vi "Login_Logout.vi"() -> ()   [LabVIEW 2020]
panel:
  in  "Tab Control":enum32{"Page 1", "Page 2", "Page 3"}(tab)
  in  "Refresh Button":bool
  in  "PassWord":string
  in  "User Name":string
  in  "Port 2":u16
  in  "Port 1":u16
  in  "Stop Send Data":bool
  in  "Send Data Button":bool
  out "Respone Led":bool
  in  "IP address":string
  in  "Export":bool caption="Export data"
  out "data":string[][](array[string]) caption="Data User"
  out "error out":errorcluster
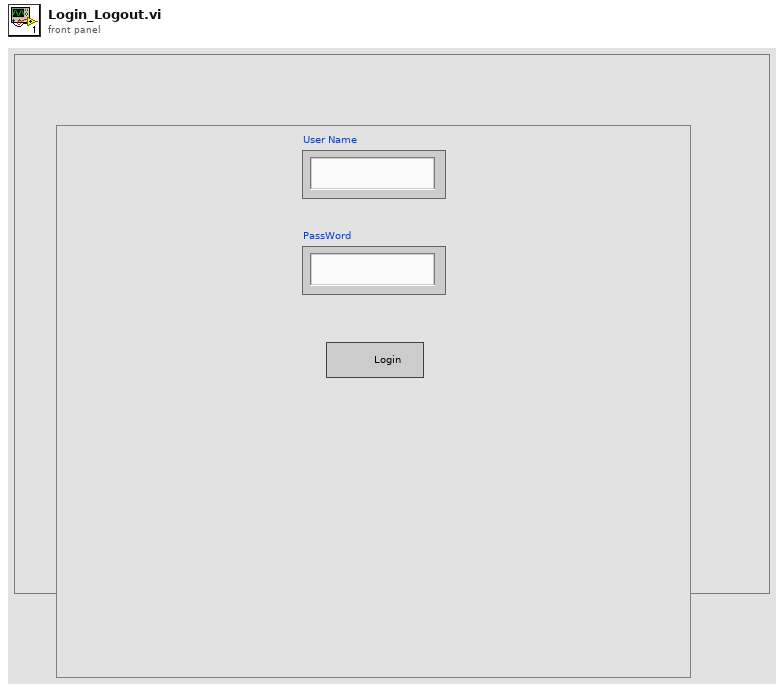
[diagram p1: front panel]
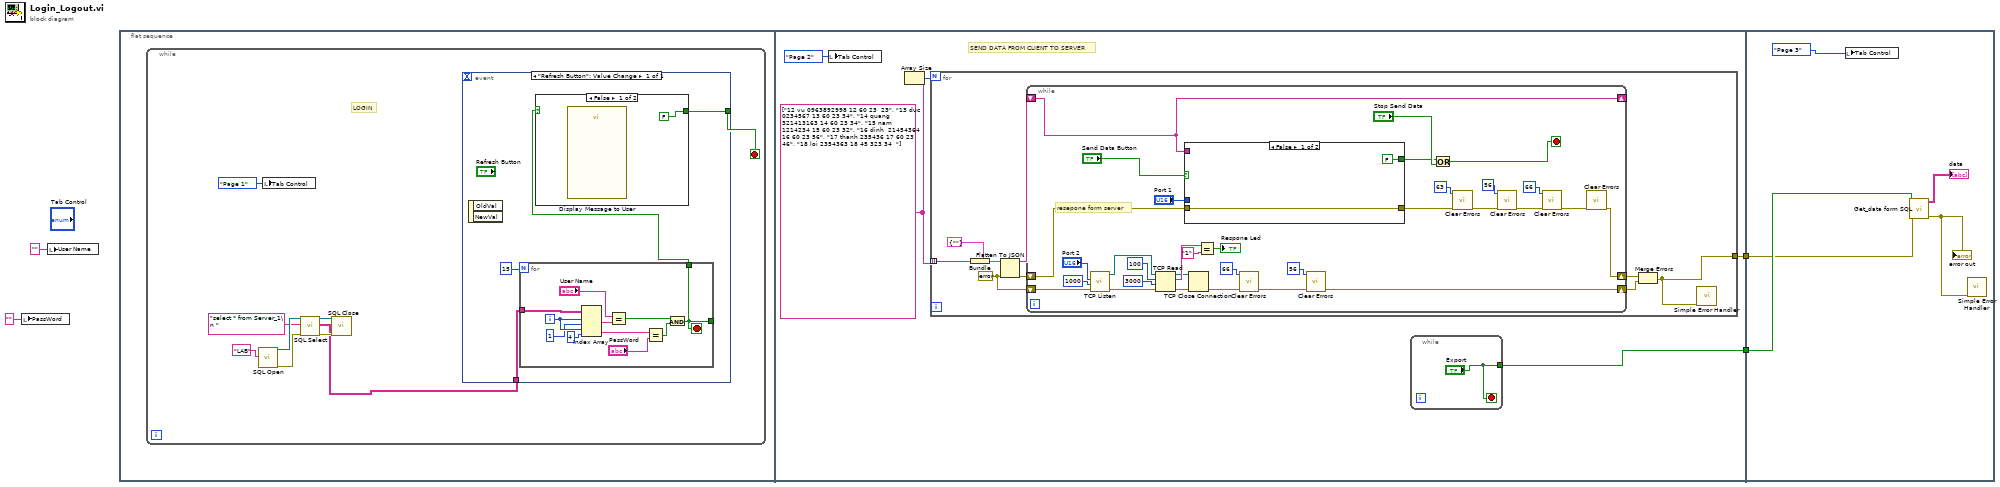
[diagram p0: block diagram]
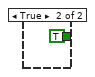
[diagram p2: hidden frame]
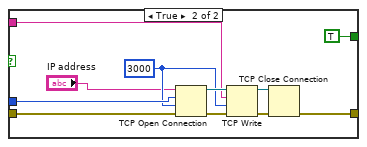
[diagram p3: hidden frame]
diagram:
  n1 = local write "PassWord"("" ("Password")) -> ()
  n2 = local write "User Name"("" ("User Name")) -> ()
  n3 = flat-sequence {
    tunnel: [w32] -> w4
    tunnel: [w31] -> w3
    tunnel: w4 -> [w93]
    tunnel: w3 -> [w92]
    frame #0 {
      n4 = while {
        stop <- w13 stop-if-true
        # "LOGIN"
        n5 = call <vilib>:"SQL Open.vi"("ConnectionString In"="LAB") -> ("Connection Out"=w9:refnum<k7>, "Error out"=w8:errorcluster)  [unwired: 17 in]
        n6 = local write "Tab Control"(enum32{"Page 1", "Page 2", "Page 3"}."Page 1" ("Tab Control")) -> ()
        n7 = call <vilib>:"SQL Select.vi"("Connection In"=w9, "SQL Query"="select * from Server_1\n ", "Error in (no error)"=w8) -> ("Connection Out"=w11:refnum<k7>, "Data"=w5:string[][], "Error out"=w10:errorcluster)  [unwired: 14 in]
        n8 = call <vilib>:"SQL Close.vi"("Connection In"=w11, "Error in (no error)"=w10) -> ()  [unwired: 17 in, 1 out]
        n9 = event shown="[0] \"Refresh Button\": Value Change" {
          selector: _ -> [_]
          dyn-events: _ -> [_]
          timeout: _ -> [_]
          tunnel: [w17] -> w13
          tunnel: w5 -> [w15]
          event "Refresh Button": Value Change {
            n10 = event-data() -> ()  [unwired: 1 in, 2 out]
            n11 = for {
              N: 15 -> [_]
              tunnel: w15 -> [w28]
              tunnel: [w18] -> _
              tunnel: [w18] -> w14
              i -> [w25]
              stop <- w18 stop-if-true
              n12 = Index Array(array=w28, index (row) #1=w25, index (col) #1=1 ("disabled index (col)"), index (row) #2=w25, index (col) #2=4 ("disabled index (col)")) -> (element #1=w27:string, element #2=w26:string)
              n13 = Equal?(x="User Name", y=w27) -> (x = y?=w21:bool)
              n14 = Equal?(x=w26, y="PassWord") -> (x = y?=w22:bool)
              n15 = And(x=w21, y=w22) -> (x .and. y?=w18:bool)
            }
            n16 = case shown="False" w14 {
              tunnel: [FALSE TRUE] -> w17
              frame False {
                n17 = call "Display Message to User"() -> ()  [unwired: 10 in, 2 out]
              }
              frame True {
              }
            }
          }
        }
      }
    }
    frame #1 {
      w34 = string[] ["12 vu 0963892998 12 60 23  23", "13 duc 0234567 13 60 23 34", "14 quang 321413163 14 60 23 34", "15 nam  1214234 15 60 23 32", "16 dinh  21454364  16 60 23 56", "17 thanh 235436 17 60 23 46", "18 loi 2354363 18 45 323 34  "]
      # "SEND DATA FROM CLIENT TO SERVER"
      n18 = local write "Tab Control"(enum32{"Page 1", "Page 2", "Page 3"}."Page 2" ("Tab Control")) -> ()
      n19 = Array Size(array=w34) -> (size(s)=w35:i32)
      n20 = for {
        N: w35 -> [_]
        tunnel: w34 -> [w42] mode=indexing
        tunnel: [w37] -> w31
        w40 = errorcluster {"status"=FALSE, "code"=0, "source"=""} ("error out")
        n21 = Bundle(cluster=cluster{"Message":string} {"Message"=""}, "Message"=w42) -> (w43:cluster{"Message":string})
        n22 = Flatten To JSON(anything=w43, error in (no error)=w40) -> (JSON string=w41:string, 11:w39:errorcluster)  [unwired: 1 in]
        n23 = while {
          shift-right: [w66] -> _
          shift-left: w41 -> [w66]
          shift-right: [w73] -> w38
          shift-left: w40 -> [w74]
          shift-right: [w49] -> w45
          shift-left: w39 -> [w72]
          stop <- w46 stop-if-true
          # "resepone form server"
          n24 = call <vilib>:"TCP Listen.vi"("error in (no error)"=w74, "timeout ms (wait forever: -1)"=1000, "port"="Port 2") -> ("error out"=w62:errorcluster, "connection ID"=w61:refnum<k5>)  [unwired: 4 in, 3 out]
          n25 = TCP Read(connection ID=w61, bytes to read=100, error in (no error)=w62, 9:3000 ("timeout ms (25000)")) -> (connection ID out=w59:refnum<k5>, data out=w76:string, error out=w60:errorcluster)  [unwired: 1 in]
          n26 = case shown="False" "Send Data Button" {
            tunnel: w66 -> [_ w86]
            tunnel: [w79 w82] -> w65
            tunnel: "Port 1" -> [_ w85]
            tunnel: w72 -> [w79 w84]
            tunnel: [FALSE TRUE] -> w55
            frame False {
            }
            frame True {
              w83 = 3000 ("timeout ms (60000)")
              n27 = TCP Open Connection(address="IP address", remote port or service name=w85, timeout ms (60000)=w83, error in (no error)=w84) -> (connection ID=w87:refnum<k5>, error out=w90:errorcluster)  [unwired: 1 in]
              n28 = TCP Write(connection ID=w87, data in=w86, error in (no error)=w90, 9:w83) -> (connection ID out=w88:refnum<k5>, error out=w89:errorcluster)  [unwired: 1 out]
              n29 = TCP Close Connection(connection ID=w88, error in (no error)=w89) -> (error out=w82:errorcluster)  [unwired: 1 in, 1 out]
            }
          }
          n30 = TCP Close Connection(connection ID=w59, error in (no error)=w60) -> (error out=w70:errorcluster)  [unwired: 1 in, 1 out]
          n31 = Equal?(x=w76, y="1") -> (x = y?=→"Respone Led":bool)
          n32 = call <vilib>:"Clear Errors.vi"("error in (no error)"=w70, "specific error code to clear (0: all)"=66) -> ("error out"=w69:errorcluster)  [unwired: 4 in, 1 out]
          n33 = call <vilib>:"Clear Errors.vi"("error in (no error)"=w69, "specific error code to clear (0: all)"=56) -> ("error out"=w73:errorcluster)  [unwired: 4 in, 1 out]
          n34 = Or(x=w55, y="Stop Send Data") -> (x .or. y?=w46:bool)
          n35 = call <vilib>:"Clear Errors.vi"("error in (no error)"=w65, "specific error code to clear (0: all)"=63) -> ("error out"=w54:errorcluster)  [unwired: 4 in, 1 out]
          n36 = call <vilib>:"Clear Errors.vi"("error in (no error)"=w54, "specific error code to clear (0: all)"=56) -> ("error out"=w52:errorcluster)  [unwired: 4 in, 1 out]
          n37 = call <vilib>:"Clear Errors.vi"("error in (no error)"=w52, "specific error code to clear (0: all)"=66) -> ("error out"=w50:errorcluster)  [unwired: 4 in, 1 out]
          n38 = call <vilib>:"Clear Errors.vi"("error in (no error)"=w50) -> ("error out"=w49:errorcluster)  [unwired: 5 in, 1 out]
        }
        n39 = Merge Errors(w45, w38) -> (w37:errorcluster)
        n40 = call <vilib>:"Simple Error Handler.vi"("error in (no error)"=w37) -> ()  [unwired: 4 in, 5 out]
      }
      n41 = while {
        tunnel: ["Export"] -> w32
        stop <- "Export" stop-if-true
      }
    }
    frame #2 {
      n42 = local write "Tab Control"(enum32{"Page 1", "Page 2", "Page 3"}."Page 3" ("Tab Control")) -> ()
      n43 = call "Get_data form SQL.vi"("error in (no error)"=w92, "Export"=w93) -> ("error out"=w94:errorcluster, "data"=→"data":string[][])  [unwired: 8 in]
      "error out" <- w94
      n44 = call <vilib>:"Simple Error Handler.vi"("error in (no error)"=w94) -> ()  [unwired: 4 in, 5 out]
    }
  }
